vi "set_clock_enabled_state.vi"(8 "error in (no error)":errorcluster, 10 "enable clocks?":bool, 11 "GenericFPGAWrapper in":refnum<class "GenericFPGAWrapper.lvclass">) -> (0 "error out":errorcluster, 3 "GenericFPGAWrapper out":refnum<class "GenericFPGAWrapper.lvclass">)   [LabVIEW 2010, in "GenericFPGAWrapper.lvclass"]
uses:
  GenericFPGAWrapper.lvclass
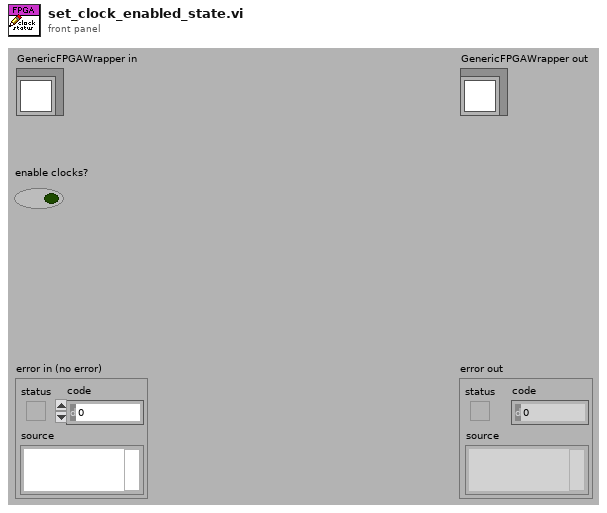
[diagram p1: front panel]
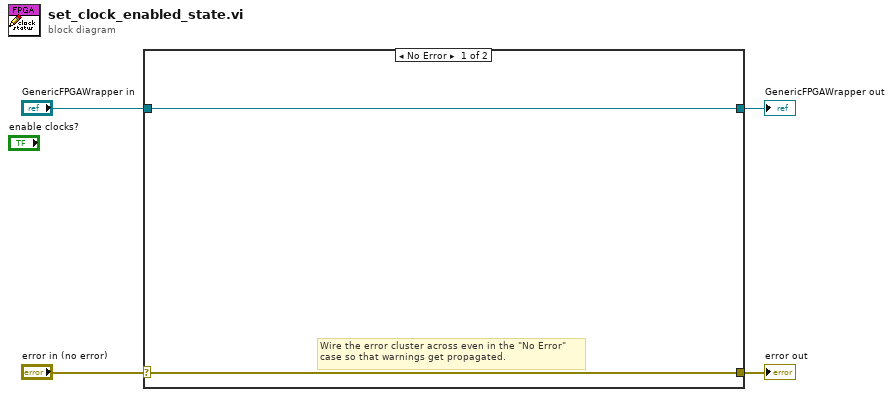
[diagram p0: block diagram]
diagram:
  n1 = case shown="No Error" "error in (no error)" {
    selector: "error in (no error)" -> [w5 w8]
    tunnel: [w5 w8] -> w3
    tunnel: [w6 w7] -> w1
    tunnel: "GenericFPGAWrapper in" -> [w6 w7]
    frame No Error {
      # "Wire the error cluster across even in the \"No Error\"\ncase so that warnings get propagated."
    }
    frame Error {
    }
  }
  "error out" <- w3
  "GenericFPGAWrapper out" <- w1
